vi "DifferentialDriveController.vi"(4 "GainsCluster":T2, 5 "prevArgIn":dbl, 6 "Setpoint Cluster":T1, 7 "prevModIn":dbl, 10 "ArgIn":dbl, 11 "ModIn":dbl) -> (1 "right motor out":dbl, 2 "left motor out":dbl)   [LabVIEW 2012]
uses:
  GainsTDef.ctl
  setpointCluster.ctl
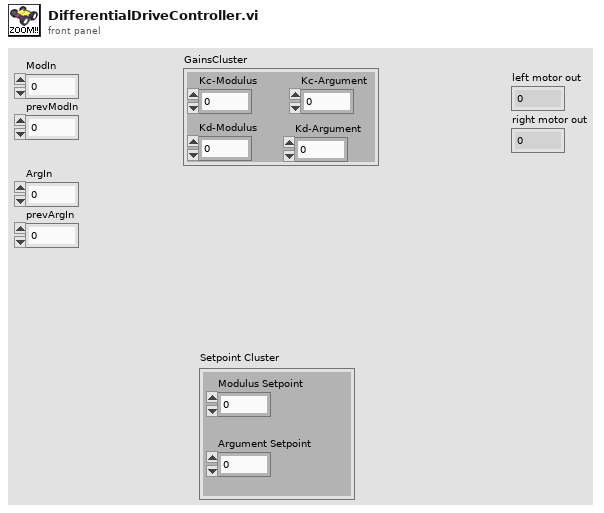
[diagram p1: front panel]
types:
  T1 = typedef "setpointCluster.ctl" = cluster{"Modulus Setpoint":dbl, "Argument Setpoint":dbl}
  T2 = typedef "GainsTDef.ctl" = cluster{"Kc-Modulus":dbl, "Kd-Modulus":dbl, "Kc-Argument":dbl, "Kd-Argument":dbl}
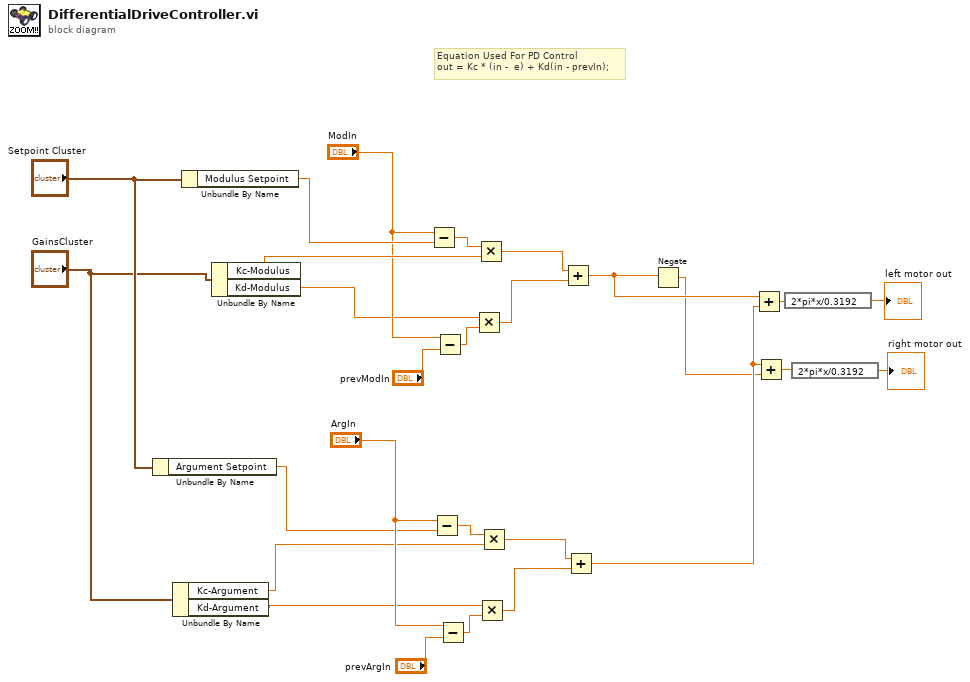
[diagram p0: block diagram]
diagram:
  # "Equation Used For PD Control\nout = Kc * (in -  e) + Kd(in - prevIn);"
  n1 = Unbundle By Name("Setpoint Cluster") -> ("Argument Setpoint"=w11:dbl)
  n2 = Unbundle By Name("GainsCluster") -> ("Kc-Argument"=w10:dbl, "Kd-Argument"=w9:dbl)
  n3 = Unbundle By Name("Setpoint Cluster") -> ("Modulus Setpoint"=w23:dbl)
  n4 = Unbundle By Name("GainsCluster") -> ("Kc-Modulus"=w24:dbl, "Kd-Modulus"=w20:dbl)
  n5 = Subtract(x="ModIn", y=w23) -> (x-y=w25:dbl)
  n6 = Subtract(x="ArgIn", y=w11) -> (x-y=w16:dbl)
  n7 = Subtract(x="ModIn", y="prevModIn") -> (x-y=w19:dbl)
  n8 = Subtract(x="ArgIn", y="prevArgIn") -> (x-y=w13:dbl)
  n9 = Multiply(x=w20, y=w19) -> (x*y=w27:dbl)
  n10 = Multiply(x=w25, y=w24) -> (x*y=w26:dbl)
  n11 = Multiply(x=w9, y=w13) -> (x*y=w18:dbl)
  n12 = Multiply(x=w16, y=w10) -> (x*y=w17:dbl)
  n13 = Add(x=w26, y=w27) -> (x+y=w8:dbl)
  n14 = Add(x=w17, y=w18) -> (x+y=w7:dbl)
  n15 = Negate(x=w8) -> (-x=w6:dbl)
  n16 = Add(x=w8, y=w7) -> (x+y=w5:dbl)
  n17 = Add(x=w7, y=w6) -> (x+y=w3:dbl)
  n18 = expression code="2*pi*x/0.3192"(w5) -> (→"left motor out":dbl)
  n19 = expression code="2*pi*x/0.3192"(w3) -> (→"right motor out":dbl)
